vi "Convert time down.vi"(10 "date time rec":T1) -> (2 "date time rec 2":T1)   [LabVIEW 2020]
uses:
  <vilib>/Utility/miscctls.llb/LVDateTimeRec.ctl
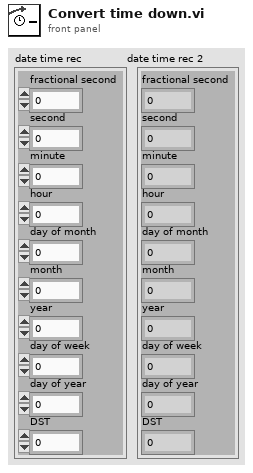
[diagram p1: front panel]
types:
  T1 = typedef "LVDateTimeRec.ctl" = cluster{"fractional second":dbl, "second":i32, "minute":i32, "hour":i32, "day of month":i32, "month":i32, "year":i32, "day of week":i32, "day of year":i32, "DST":i32}
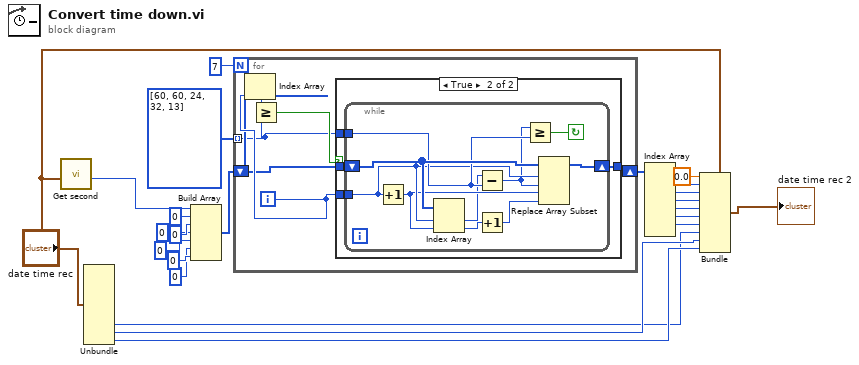
[diagram p0: block diagram]
diagram:
  n1 = call "Get second.vi"("date time rec"="date time rec") -> ("output variable"=w11:i32)  [unwired: 10 in]
  n2 = Unbundle("date time rec") -> ("day of week"=w2:i32, "day of year"=w3:i32, "DST"=w4:i32)  [unwired: 7 out]
  n3 = Build Array(w11, 0 ("element"), 0 ("element"), 0 ("element"), 0 ("element"), 0 ("element"), 0 ("element")) -> (w22:i32[])
  n4 = for {
    N: 7 -> [_]
    tunnel: i32[] [60, 60, 24, 32, 13] -> [w24] mode=indexing
    shift-right: [w29] -> w20
    shift-left: w22 -> [w26]
    i -> [w27]
    n5 = Index Array(array=w26, index=w27) -> (element=w25:i32)
    n6 = Greater Or Equal?(x=w25, y=w24) -> (x >= y?=w28:bool)
    n7 = case shown="True" w28 {
      tunnel: w24 -> [_ w34]
      tunnel: w27 -> [_ w33]
      tunnel: w26 -> [w30 w32]
      tunnel: [w30 w31] -> w29
      frame False {
      }
      frame True {
        n8 = while {
          tunnel: w34 -> [w41]
          tunnel: w33 -> [w40]
          shift-right: [w43] -> w31
          shift-left: w32 -> [w42]
          stop <- w44 continue-if-true
          n9 = Increment(x=w40) -> (x+1=w39:i32)
          n10 = Index Array(array=w42, index #1=w40, index #2=w39) -> (element #1=w36:i32, element #2=w38:i32)
          n11 = Subtract(x=w36, y=w41) -> (x-y=w35:i32)
          n12 = Increment(x=w38) -> (x+1=w37:i32)
          n13 = Greater Or Equal?(x=w35, y=w41) -> (x >= y?=w44:bool)
          n14 = Replace Array Subset(array=w42, new element #1=w35, index #1=w40, new element #2=w37, index #2=w39) -> (w43:i32[])
        }
      }
    }
  }
  n15 = Index Array(array=w20) -> (element #1=w19:i32, element #2=w18:i32, element #3=w17:i32, element #4=w16:i32, element #5=w15:i32, element #6=w14:i32)  [unwired: 7 in, 1 out]
  n16 = Bundle(cluster="date time rec", "fractional second"=0.0, "second"=w19, "minute"=w18, "hour"=w17, "day of month"=w16, "month"=w15, "year"=w14, "day of week"=w2, "day of year"=w3, "DST"=w4) -> (→"date time rec 2":T1)
